vi "fix class control labels.vi"(8 "error in":errorcluster, 10 "class to load":path, 11 "Application in":refnum<vi>) -> (0 "error out":errorcluster)   [LabVIEW 2013, in "DCAFConfigurablePluginDecideFeatures.lvclass"]
uses:
  DCAFConfigurablePluginDecideFeatures.lvclass
  <vilib>/Utility/traverseref.llb/TRef TravTarget.ctl
  <vilib>/Utility/traverseref.llb/VI Scripting - Traverse.lvlib
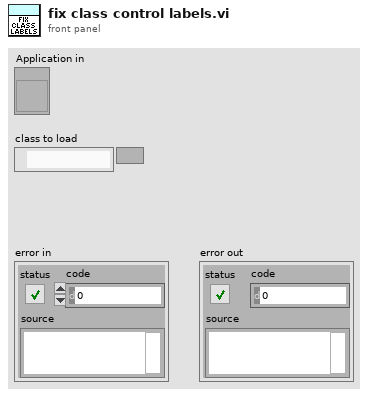
[diagram p1: front panel]
types:
  T1 = typedef "TRef TravTarget.ctl" = enum16{"FP", "BD", "Other"}
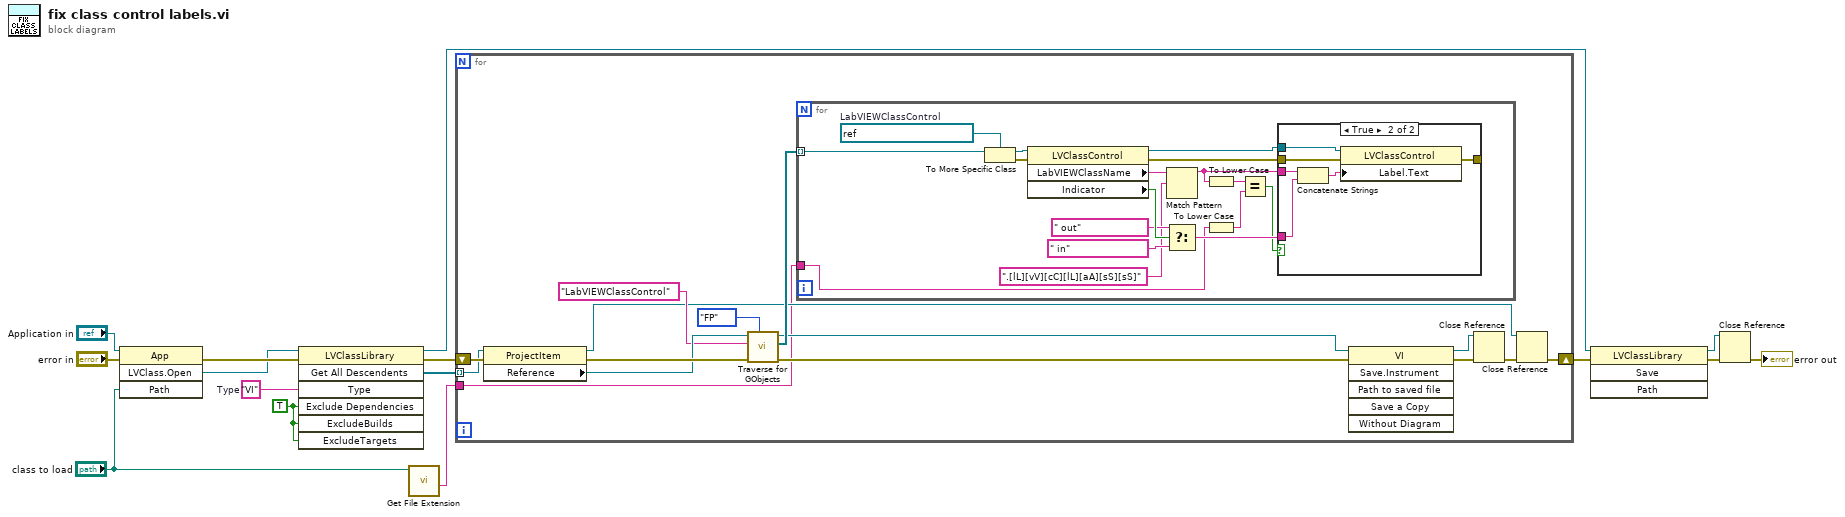
[diagram p0: block diagram]
diagram:
  w11 = TRUE
  w10 = "VI"  # Type
  n1 = invoke class="App" method="LVClass.Open"(reference="Application in", error in="error in", "Path"="class to load") -> (error out=w12:errorcluster, "LVClass.Open"=w9:refnum<vi>)  [unwired: 1 in, 2 out]
  n2 = invoke class="LVClassLibrary" method="Get All Descendents"(reference=w9, error in=w12, "Type"=w10, "Exclude Dependencies"=w11, "ExcludeBuilds"=w11, "ExcludeTargets"=w11) -> (reference out=w7:refnum<vi>, error out=w14:errorcluster, "All Descendents"=w13:refnum<vi>[])  [unwired: 1 in, 4 out]
  n3 = call <vilib>:"Get File Extension.vi"("file"="class to load") -> ("filename without extension"=w1:string)  [unwired: 7 in, 3 out]
  n4 = for {
    tunnel: w13 -> [w29] mode=indexing
    shift-right: [w21] -> w15
    shift-left: w14 -> [w30]
    tunnel: w1 -> [w16]
    n5 = property class="ProjectItem"(reference=w29, error in=w30) -> (reference out=w20:refnum<vi>, error out=w28:errorcluster, "Reference"=w27:refnum<vi>)
    n6 = call <vilib>:"Traverse for GObjects.vi"("Traverse Target"=TRef_TravTarget."FP", "error in (no error)"=w28, "Class Name"="LabVIEWClassControl", "VI Refnum"=w27) -> ("error out"=w17:errorcluster, "References"=w24:refnum<vi>[], "dup VI Refnum"=w23:refnum<vi>)  [unwired: 4 in, 1 out]
    n7 = for {
      tunnel: w24 -> [w46] mode=indexing
      tunnel: w16 -> [w35]
      w44 = refnum<vi> refnum  # LabVIEWClassControl
      n8 = To More Specific Class(target class=w44, reference=w46) -> (specific class reference=w45:refnum<vi>, error out=w47:errorcluster)  [unwired: 1 in]
      n9 = property class="LVClassControl"(reference=w45, error in=w47) -> (reference out=w43:refnum<vi>, error out=w42:errorcluster, "LabVIEWClassName"=w37:string, "Indicator"=w41:bool)
      n10 = Match Pattern(string=w37, regular expression=".[lL][vV][cC][lL][aA][sS][sS]") -> (before substring=w34:string)  [unwired: 1 in, 3 out]
      n11 = Select(t=" out", s=w41, f=" in") -> (s? t:f=w38:string)
      n12 = To Lower Case(string=w34) -> (all lower case string=w32:string)
      n13 = To Lower Case(string=w35) -> (all lower case string=w33:string)
      n14 = Equal?(x=w32, y=w33) -> (x = y?=w31:bool)
      n15 = case shown="True" w31 {
        tunnel: w43 -> [_ w54]
        tunnel: w42 -> [w48 w53]
        tunnel: w38 -> [_ w51]
        tunnel: [w48 w50] -> _
        tunnel: w34 -> [_ w49]
        frame False {
        }
        frame True {
          n16 = Concatenate Strings(w49, w51) -> (w52:string)
          n17 = property class="LVClassControl"(reference=w54, error in=w53, "Label.Text"=w52) -> (error out=w50:errorcluster)  [unwired: 1 out]
        }
      }
    }
    n18 = invoke class="VI" method="Save.Instrument"(reference=w23, error in=w17) -> (reference out=w18:refnum<vi>, error out=w19:errorcluster)  [unwired: 4 in, 4 out]
    n19 = Close Reference(reference=w18, error in (no error)=w19) -> (error out=w22:errorcluster)
    n20 = Close Reference(reference=w20, error in (no error)=w22) -> (error out=w21:errorcluster)
  }
  n21 = invoke class="LVClassLibrary" method="Save"(reference=w7, error in=w15) -> (reference out=w6:refnum<vi>, error out=w8:errorcluster)  [unwired: 2 in, 2 out]
  n22 = Close Reference(reference=w6, error in (no error)=w8) -> (error out=→"error out":errorcluster)
